vi "LOC ReTx Delay.vi"(0 "Last Valid In":u32, 5 "ReTxDelay":u32, 7 "Ping Time Out?":bool) -> (11 "Last Valid Out":u32)   [LabVIEW 2018]
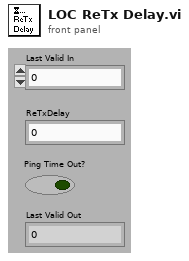
[diagram p1: front panel]
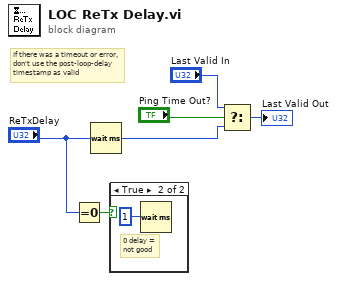
[diagram p0: block diagram]
diagram:
  # "If there was a timeout or error,\ndon't use the post-loop-delay \ntimestamp as valid"
  n1 = Equal To 0?(x="ReTxDelay") -> (x = 0?=w5:bool)
  n2 = Wait (ms)(milliseconds to wait="ReTxDelay") -> (millisecond timer value=w2:u32)
  n3 = case shown="True" w5 {
    frame False {
    }
    frame True {
      # "0 delay = \nnot good"
      n4 = Wait (ms)(milliseconds to wait=u32 1) -> ()  [unwired: 1 out]
    }
  }
  n5 = Select(t="Last Valid In", s="Ping Time Out?", f=w2) -> (s? t:f=→"Last Valid Out":u32)
